vi "Static.vi"() -> ()   [LabVIEW 2017, in "MGI-Panel Manager.lvlib" / "Panel Registry.lvclass"]
uses:
  Panel Registry.lvclass
panel:
  out "Last Event":variant
  out "Panel State":variant
  out "Event Lookup":variant
  out "Parent Lookup":variant
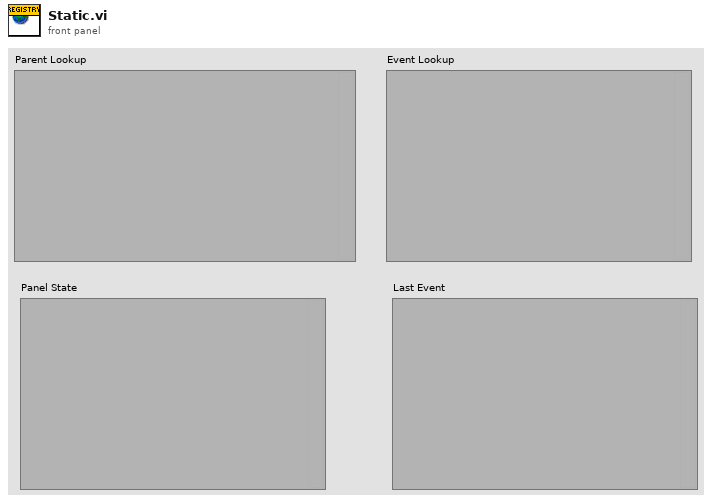
[diagram p1: front panel]
diagram:
